vi "Motic Get Gain List.vi"(8 "error in (no error)":errorcluster, 10 "gain count":i32, 11 "camera":i32) -> (0 "error out":errorcluster, 1 "max gain":sgl, 2 "gain list array out":sgl[](array[numeric]), 3 "camera out":i32, 4 "min gain":sgl)   [LabVIEW 2012, in "MoticApi.lvlib"]
doc: "MOTICAPI bool Motic_GetGainList(MUCam_Handle camera, float *g);"
uses:
  MoticApi.lvlib
  MoticApi.dll
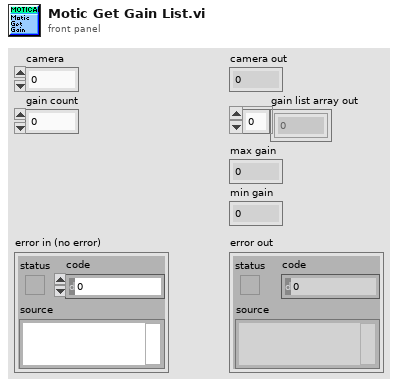
[diagram p1: front panel]
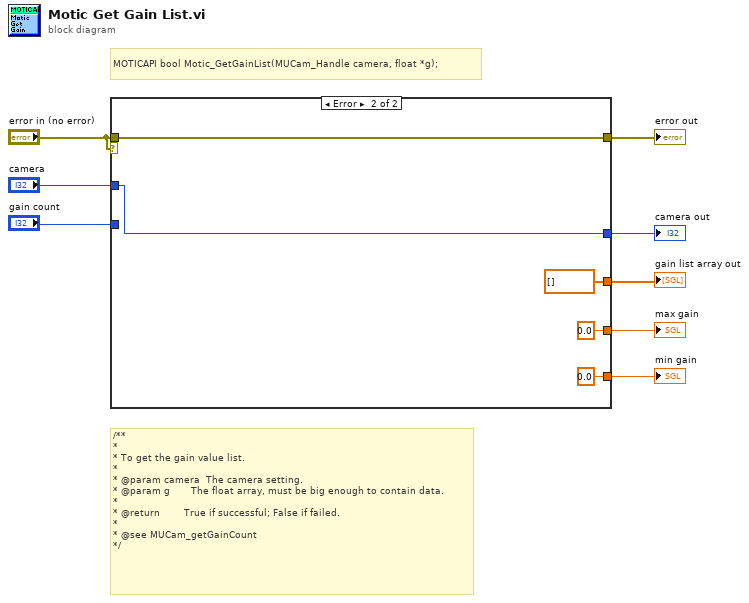
[diagram p0: block diagram]
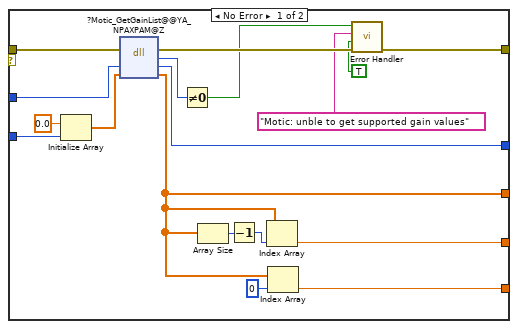
[diagram p2: hidden frame]
diagram:
  # "/**\n*\n* To get the gain value list.\n*\n* @param camera  The camera setting.\n* @param g       The float array, must be big enough to contain data.\n*\n* @return        True if successful; False if failed.\n*\n* @see MUCam_getGainCount\n*/"
  # "MOTICAPI bool Motic_GetGainList(MUCam_Handle camera, float *g);"
  n1 = case shown="Error" "error in (no error)" {
    tunnel: "camera" -> [w25 w30]
    tunnel: [w24 w30] -> w7
    tunnel: "error in (no error)" -> [w23 w31]
    tunnel: [w22 w31] -> w6
    tunnel: "gain count" -> [w16 _]
    tunnel: [w12 sgl 0.0] -> w4
    tunnel: [w11 sgl[] [] ("gain list array out")] -> w3
    tunnel: [w9 sgl 0.0] -> w2
    frame No Error {
      n2 = Initialize Array(sgl 0.0 ("element"), w16) -> (w15:sgl[])
      n3 = dll-call lib="C:/Users/TTS-Digital/Desktop/MoticApi/MoticApi_git/MoticApi/MoticApi.*" fn="?Motic_GetGainList@@YA_NPAXPAM@Z"(error in=w23, "camera"=w25, "gain list array out"=w15) -> (error out=w21:errorcluster, "return type"=w26:u8, "camera"=w24:i32, "gain list array out"=w11:sgl[])  [unwired: 2 in, 1 out]
      n4 = Not Equal To 0?(x=w26) -> (x != 0?=w20:bool)
      n5 = Array Size(array=w11) -> (size(s)=w14:i32)
      n6 = Decrement(x=w14) -> (x-1=w13:i32)
      n7 = Index Array(array=w11, index=w13) -> (element=w12:sgl)
      n8 = Index Array(array=w11, index=0) -> (element=w9:sgl)
      n9 = call "Error Handler.vi"("error in (no error)"=w21, "Is warning?"=TRUE, "Error message"="Motic: unble to get supported gain values", "Function return"=w20) -> ("error out"=w22:errorcluster)  [unwired: 7 in]
    }
    frame Error {
    }
  }
  "camera out" <- w7
  "error out" <- w6
  "gain list array out" <- w3
  "max gain" <- w4
  "min gain" <- w2
